vi "RobotStatus.vi"(0 "Universal Robot.lvclass in":refnum<class "Universal Robot.lvclass">, 5 "error in (no error)":errorcluster) -> (14 "Universal Robot.lvclass out":refnum<class "Universal Robot.lvclass">, 15 "Robot Status":T1, 19 "error out":errorcluster)   [LabVIEW 2016, in "Universal Robot.lvclass"]
uses:
  Universal Robot.lvclass
  RobotStatus.ctl
  RobotMode.ctl
  OperationalMode.ctl
  SafetyStatus.ctl
  Universal Robot.lvclass/Universal Robot.ctl
  DashboardServer/Dashboard Server.lvclass
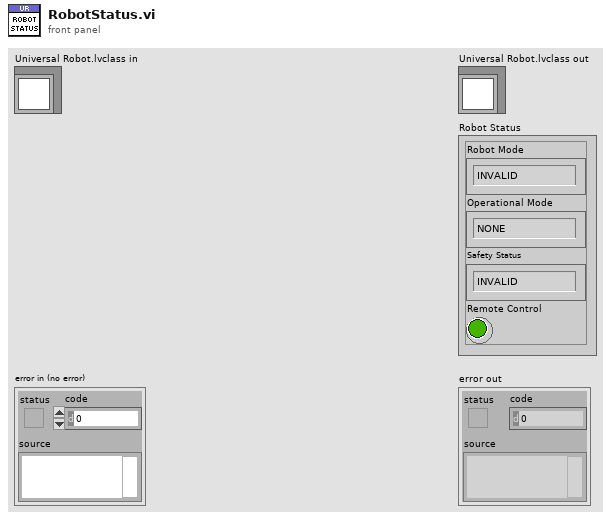
[diagram p1: front panel]
types:
  T1 = typedef "Universal Robot.lvclass/RobotStatus.ctl" = cluster{"Robot Mode":T2, "Operational Mode":T3, "Safety Status":T4, "Remote Control":bool}
  T2 = typedef "Universal Robot.lvclass/RobotMode.ctl" = enum16{"INVALID", "NO_CONTROLLER", "DISCONNECTED", "CONFIRM_SAFETY", "BOOTING", "POWER_OFF", "POWER_ON", "IDLE", "BACKDRIVE", "RUNNING"}
  T3 = typedef "Universal Robot.lvclass/OperationalMode.ctl" = enum16{"NONE", "MANUAL", "AUTOMATIC"}
  T4 = typedef "Universal Robot.lvclass/SafetyStatus.ctl" = enum16{"INVALID", "NORMAL", "REDUCED", "PROTECTIVE_STOP", "RECOVERY", "SAFEGAURD_STOP", "SYSTEM_EMERGENCY_STOP", "ROBOT_EMERGENCY_STOP", "VIOLATION", "FAULT", "AUTOMATIC_MODE_SAFEGAURD_STOP", "SYSTEM_THREE_POSITION_ENABLING_STOP"}
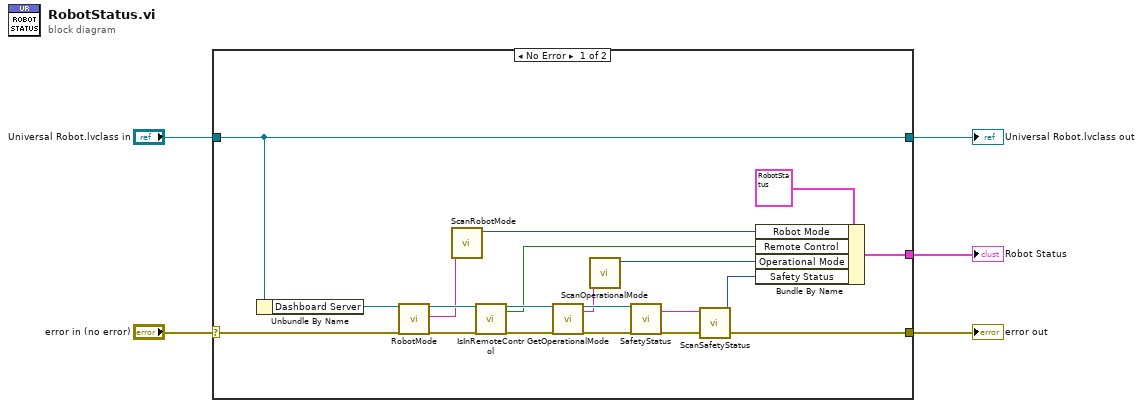
[diagram p0: block diagram]
diagram:
  n1 = case shown="No Error" "error in (no error)" {
    selector: "error in (no error)" -> [w23 w26]
    tunnel: [w18 w26] -> w4
    tunnel: "Universal Robot.lvclass in" -> [w24 w25]
    tunnel: [w24 w25] -> w2
    tunnel: [w11 _] -> w1
    frame No Error {
      n2 = Unbundle By Name(w24) -> ("Dashboard Server"=w22:refnum<class "Dashboard Server.lvclass">)
      n3 = call-dynamic "RobotMode.vi"("DashboardServer in"=w22, "error in (no error)"=w23) -> ("DashboardServer out"=w21:refnum<class "Dashboard Server.lvclass">, "robotMode"=w6:string, "error out"=w17:errorcluster)  [unwired: 15 in]
      n4 = call "ScanRobotMode.vi"("robotMode in"=w6) -> ("robotMode out"=w13:T2)  [unwired: 10 in]
      n5 = call-dynamic "IsInRemoteControl.vi"("DashboardServer in"=w21, "error in (no error)"=w17) -> ("DashboardServer out"=w20:refnum<class "Dashboard Server.lvclass">, "remoteControl"=w12:bool, "error out"=w16:errorcluster)  [unwired: 15 in]
      n6 = call-dynamic "GetOperationalMode.vi"("DashboardServer in"=w20, "error in (no error)"=w16) -> ("DashboardServer out"=w19:refnum<class "Dashboard Server.lvclass">, "operationalMode"=w10:string, "error out"=w15:errorcluster)  [unwired: 15 in]
      n7 = call "ScanOperationalMode.vi"("operationalMode in"=w10) -> ("operationalMode out"=w9:T3)  [unwired: 10 in]
      n8 = call-dynamic "SafetyStatus.vi"("DashboardServer in"=w19, "error in (no error)"=w15) -> ("safetyStatus"=w8:string, "error out"=w18:errorcluster)  [unwired: 15 in, 1 out]
      n9 = call "ScanSafetyStatus.vi"("safetyStatus in"=w8) -> ("safetyStatus out"=w7:T4)  [unwired: 10 in]
      n10 = Bundle By Name(cluster=T1 {"Robot Mode"=enum."INVALID", "Operational Mode"=enum."NONE", "Safety Status"=enum."INVALID", "Remote Control"=FALSE} ("Robot Status"), "Robot Mode"=w13, "Remote Control"=w12, "Operational Mode"=w9, "Safety Status"=w7) -> (w11:T1)
    }
    frame Error {
    }
  }
  "error out" <- w4
  "Universal Robot.lvclass out" <- w2
  "Robot Status" <- w1
